vi "run.vi"(8 "error in (no error)":errorcluster, 11 "DL090503StimulatorScaffold in":refnum<class "StimulatorDL090503.lvclass">) -> (0 "error out":errorcluster, 3 "DL090503StimulatorScaffold out":refnum<class "StimulatorDL090503.lvclass">)   [LabVIEW 2010, in "StimulatorDL090503.lvclass"]
uses:
  StimulatorDL090503.lvclass
  pattern_type_enum.ctl
  common/xcontrols/XSettings/XSettings/XSettings.xctl
  common/classes/GenericComponent/GenericComponent/GenericComponent.lvclass
  main/labview_source/controls/undock_button.ctl
  StimulatorDL090503.lvclass/StimulatorDL090503.ctl
  StimulatorDL090503Scaffold/StimulatorDL090503Scaffold/StimulatorDL090503Scaffold.lvclass
  common/classes/ErrorController/ErrorController/class_data.vi
  GenericStimulator/GenericStimulator/GenericStimulator.lvclass
  common/classes/ErrorController/ErrorController/ErrorController.lvclass
panel:
  in  "button:undock":T1
  in  "Tab Control":enum32{"User", "Debug", "About"}(tab)
  in  "temp offset":dbl=1.0 caption="offset"
  in  "duration":dbl[unit]=1.0
  in  "test":bool
  in  "offset":dbl[unit]
  in  "repetition period":dbl[unit]=1.0
  in  "repetitions":i32=1
  out "stimulating?":bool
  in  "frequency":dbl[unit]=1.0
  in  "amplitude":dbl=1.0
  in  "XSettings":refnum<class "GenericComponent.lvclass">(xcontrol)
  in  "pattern":T2
  out "finished?":bool=TRUE
  out "loaded settings?":bool
  # "pattern"
  # "application"
  # "StimulatorDL090503\n\nImplemented by:\nDominik Langer, University of Zurich"
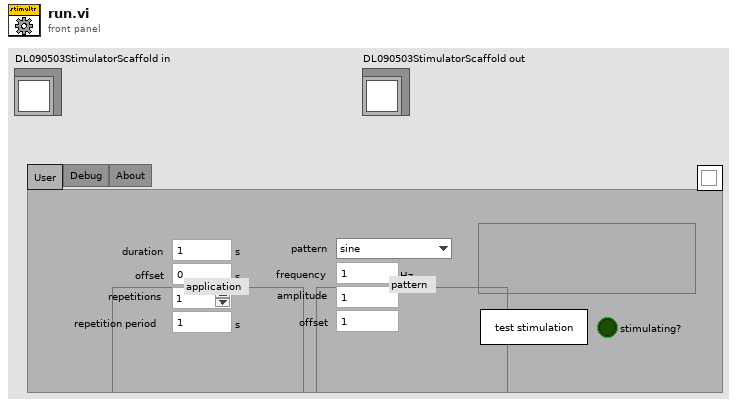
[diagram p1: front panel]
types:
  T1 = typedef "undock_button.ctl" = bool
  T2 = typedef "StimulatorDL090503.lvclass/pattern_type_enum.ctl" = enum16{"sine", "square (+/-)", "square (+)", "square (-)"}
  T3 = typedef "GenericToplevelComponent.lvclass/common_trigger_enum.ctl" = enum16{"NULL", "initialise", "terminate", "fetch command", "fetch data", "attach observer", "register as observer", "detach observer", "acknowledge", "start", "stop", "sweep started", "sweep finished", "experiment started", "experiment stopped"}
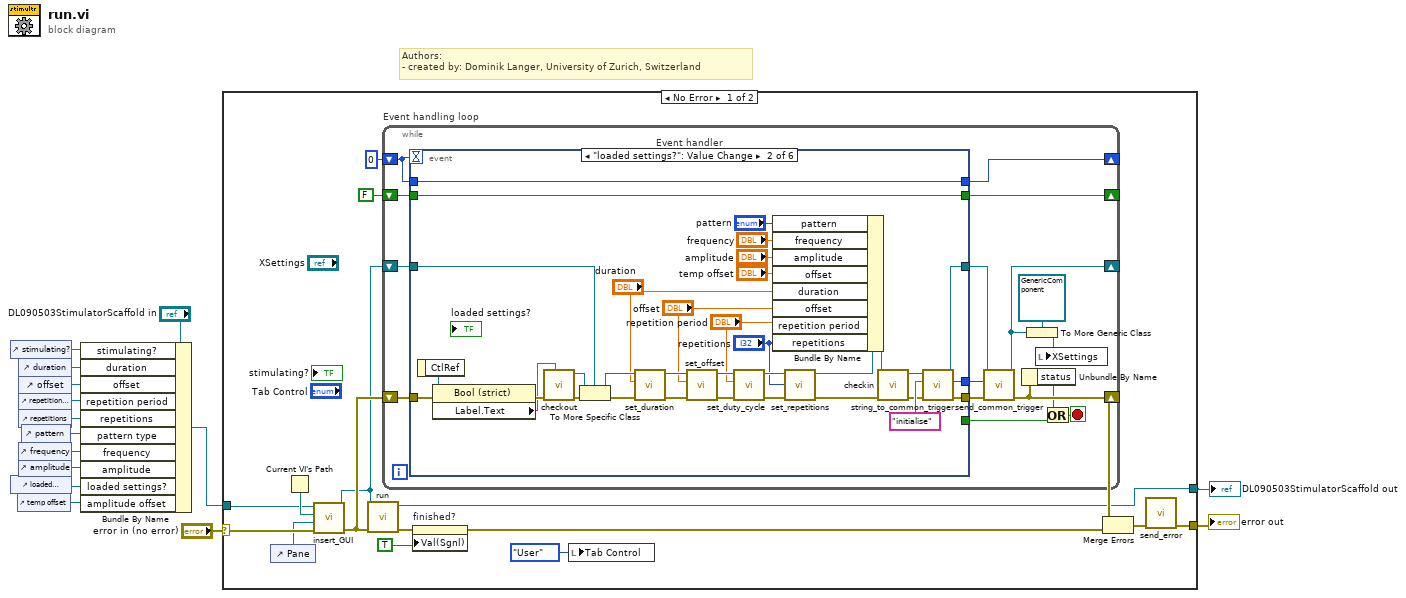
[diagram p0: block diagram]
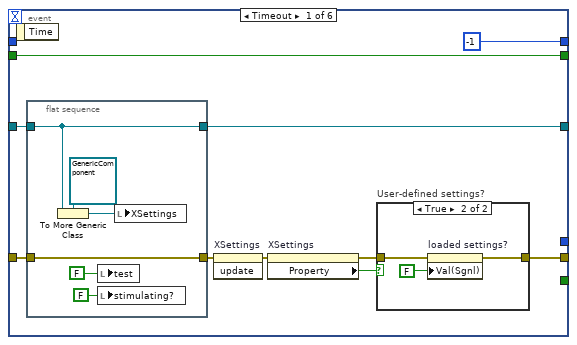
[diagram p2: hidden frame]
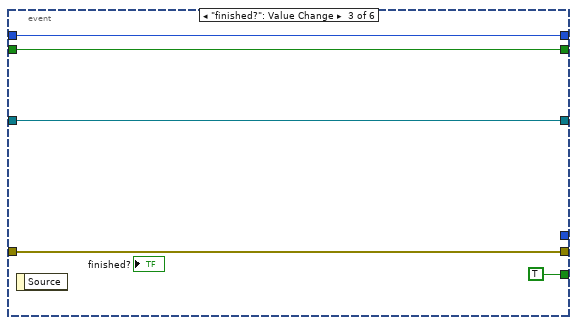
[diagram p4: hidden frame]
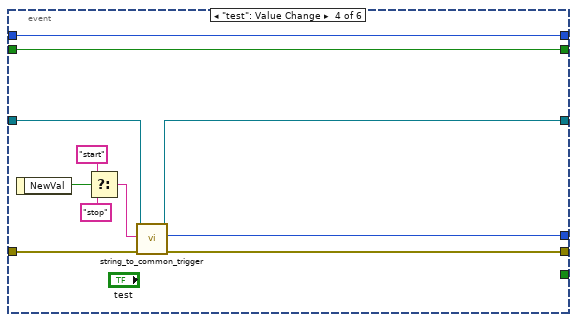
[diagram p5: hidden frame]
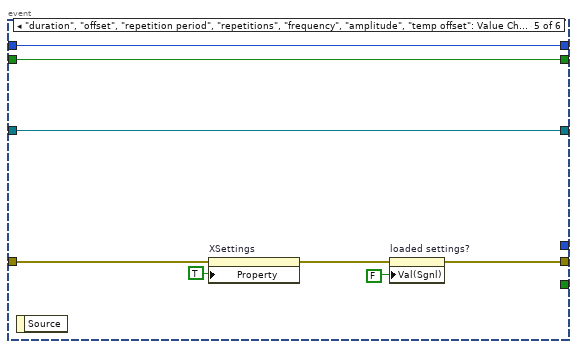
[diagram p6: hidden frame]
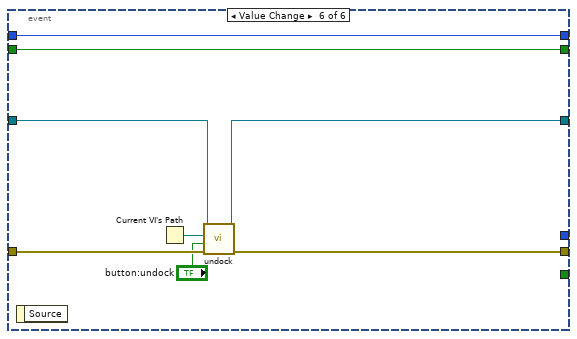
[diagram p7: hidden frame]
diagram:
  # "Authors: \n- created by: Dominik Langer, University of Zurich, Switzerland"
  n1 = control-ref of="stimulating?"() -> (w14:refnum<vi>)
  n2 = control-ref of="loaded settings?"() -> (w7:refnum<vi>)
  n3 = control-ref of="temp offset"() -> (w6:refnum<vi>)
  n4 = control-ref of="duration"() -> (w13:refnum<vi>)
  n5 = control-ref of="offset"() -> (w12:refnum<vi>)
  n6 = control-ref of="repetition period"() -> (w11:refnum<vi>)
  n7 = control-ref of="repetitions"() -> (w10:refnum<vi>)
  n8 = control-ref of="frequency"() -> (w9:refnum<vi>)
  n9 = control-ref of="amplitude"() -> (w8:refnum<vi>)
  n10 = control-ref of="pattern"() -> (w1:refnum<vi>)
  n11 = Bundle By Name(cluster="DL090503StimulatorScaffold in", "stimulating?"=w14, "duration"=w13, "offset"=w12, "repetition period"=w11, "repetitions"=w10, "pattern type"=w1, "frequency"=w9, "amplitude"=w8, "loaded settings?"=w7, "amplitude offset"=w6) -> (w15:refnum<class "StimulatorDL090503.lvclass">)
  n12 = case shown="No Error" "error in (no error)" {
    selector: "error in (no error)" -> [w22 w134]
    tunnel: [w18 w134] -> w4
    tunnel: w15 -> [w21 w135]
    tunnel: [w17 w135] -> w3
    frame No Error {
      n13 = control-ref of="Pane"() -> (w16:refnum<vi>)
      n14 = Current VI's Path() -> (path=w25:path)
      n15 = call-dynamic "insert_GUI.vi"("error in (no error)"=w22, "Pane"=w16, "VI path"=w25, "GenericComponent in"=w21) -> ("error out"=w26:errorcluster, "GenericComponent out"=w24:refnum<class "StimulatorDL090503.lvclass">)  [unwired: 6 in]
      n16 = call-parent "run.vi"("error in (no error)"=w26, "DL090503StimulatorScaffold in"=w24) -> ("error out"=w27:errorcluster, "DL090503StimulatorScaffold out"=w17:refnum<class "StimulatorDL090503.lvclass">)  [unwired: 8 out]
      n17 = while "Event handling loop" {
        shift-right: [w45] -> _
        shift-left: 0 -> [w46]
        shift-right: [w36] -> _
        shift-left: FALSE -> [w37]
        shift-right: [w41] -> w31
        shift-left: w26 -> [w47]
        shift-right: [w32] -> _
        shift-left: w24 -> [w44]
        stop <- w38 stop-if-true
        n18 = event "Event handler" shown="[1] \"loaded settings?\": Value Change" {
          selector: _ -> [_ _ _ _ _ _]
          dyn-events: _ -> [_ _ _ _ _ _]
          timeout: w46 -> [_ _ _ _ _ _]
          tunnel: w47 -> [w54 w98 w106 w114 w118 w131]
          tunnel: [w49 w76 w106 w113 w119 w130] -> w43
          tunnel: [_ _ TRUE _ _ _] -> w40
          tunnel: [-1 w101 w102 w117 w125 w133] -> w45
          tunnel: w46 -> [_ w101 w102 w117 w125 w133]
          tunnel: w44 -> [w55 w75 w104 w112 w122 w129]
          tunnel: [w53 w74 w104 w111 w122 w128] -> w34
          tunnel: [_ w71 _ w110 _ _] -> w42
          tunnel: w37 -> [w56 w100 w103 w116 w124 w132]
          tunnel: [w56 w100 w103 w116 w124 w132] -> w36
          event Timeout {
            n19 = event-data() -> ()  [unwired: 2 out]
            n20 = flat-sequence {
              tunnel: w55 -> [w63]
              tunnel: w54 -> [w62]
              tunnel: [w63] -> w53
              tunnel: [w62] -> w52
              frame #0 {
                n21 = To More Generic Class(target class=refnum<class "GenericComponent.lvclass"> refnum ("GenericComponent.lvclass"), reference=w63) -> (generic class reference=w65:refnum<class "GenericComponent.lvclass">)
                n22 = local write "test"(FALSE ("test")) -> ()
                n23 = local write "stimulating?"(FALSE ("stimulating?")) -> ()
                n24 = local write "XSettings"(w65) -> ()
              }
            }
            n25 = invoke on="XSettings" class="XSettings (strict)" method="update"(error in=w52) -> (error out=w51:errorcluster)  [unwired: 2 in, 2 out]
            n26 = property on="XSettings" class="XSettings (strict)"(error in=w51) -> (error out=w50:errorcluster, "Property"=w48:bool)  [unwired: 1 in, 1 out]
            n27 = case "User-defined settings?" shown="True" w48 {
              tunnel: w50 -> [w58 w60]
              tunnel: [w58 w59] -> w49
              frame False {
              }
              frame True {
                n28 = property on="loaded settings?" class="Bool (strict)"(error in=w60, "Val(Sgnl)"=FALSE) -> (error out=w59:errorcluster)  [unwired: 1 in, 1 out]
              }
            }
          }
          event "loaded settings?": Value Change {
            n29 = event-data() -> ("CtlRef"=w99:refnum<vi>)  [unwired: 1 out]
            n30 = property class="Bool (strict)"(reference=w99, error in=w98) -> (error out=w77:errorcluster, "Label.Text"=w72:string)  [unwired: 1 out]
            n31 = call "checkout.vi"("locked by?"=w72, "error in (no error)"=w77) -> ("error out"=w97:errorcluster, "GenericStimulator out"=w96:refnum<class "GenericStimulator.lvclass">)  [unwired: 8 out]
            n32 = To More Specific Class(target class=w75, reference=w96, error in=w97) -> (specific class reference=w95:refnum<class "StimulatorDL090503.lvclass">, error out=w94:errorcluster)
            n33 = call-dynamic "set_duration.vi"("error in (no error)"=w94, "duration"="duration", "DL090503StimulatorScaffold.lvclass in"=w95) -> ("error out"=w90:errorcluster, "DL090503StimulatorScaffold.lvclass out"=w88:refnum<class "StimulatorDL090503.lvclass">)  [unwired: 7 out]
            n34 = call-dynamic "set_offset.vi"("error in (no error)"=w90, "offset"="offset", "DL090503StimulatorScaffold.lvclass in"=w88) -> ("error out"=w89:errorcluster, "DL090503StimulatorScaffold.lvclass out"=w87:refnum<class "StimulatorDL090503.lvclass">)  [unwired: 7 out]
            n35 = call-dynamic "set_duty_cycle.vi"("error in (no error)"=w89, "duty cycle"="repetition period", "DL090503StimulatorScaffold.lvclass in"=w87) -> ("error out"=w92:errorcluster, "DL090503StimulatorScaffold.lvclass out"=w91:refnum<class "StimulatorDL090503.lvclass">)  [unwired: 7 out]
            n36 = call-dynamic "set_repetitions.vi"("error in (no error)"=w92, "repetitions"="repetitions", "DL090503StimulatorScaffold.lvclass in"=w91) -> ("error out"=w93:errorcluster, "DL090503StimulatorScaffold.lvclass out"=w82:refnum<class "StimulatorDL090503.lvclass">)  [unwired: 7 out]
            n37 = Bundle By Name(cluster=w82, "pattern"="pattern", "frequency"="frequency", "amplitude"="amplitude", "offset"="temp offset", "duration"="duration", "offset"="offset", "repetition period"="repetition period", "repetitions"="repetitions") -> (w81:refnum<class "StimulatorDL090503.lvclass">)
            n38 = call-dynamic "checkin.vi"("error in (no error)"=w93, "GenericStimulator in"=w81) -> ("error out"=w79:errorcluster, "GenericStimulator out"=w78:refnum<class "StimulatorDL090503.lvclass">)  [unwired: 8 in]
            n39 = call-dynamic "string_to_common_trigger.vi"("error in (no error)"=w79, "trigger string"="initialise", "GenericToplevelComponent in"=w78) -> ("error out"=w76:errorcluster, "trigger"=w71:T3, "GenericToplevelComponent out"=w74:refnum<class "StimulatorDL090503.lvclass">)  [unwired: 6 in]
          }
          event "finished?": Value Change {
            n40 = event-data() -> ()  [unwired: 2 out]
          }
          event "test": Value Change {
            n41 = event-data() -> ("NewVal"=w115:bool)  [unwired: 1 out]
            n42 = Select(t="start", s=w115, f="stop") -> (s? t:f=w109:string)
            n43 = call-dynamic "string_to_common_trigger.vi"("error in (no error)"=w114, "trigger string"=w109, "GenericToplevelComponent in"=w112) -> ("error out"=w113:errorcluster, "trigger"=w110:T3, "GenericToplevelComponent out"=w111:refnum<class "StimulatorDL090503.lvclass">)  [unwired: 6 in]
          }
          event "duration", "offset", "repetition period", "repetitions", "frequency", "amplitude", "temp offset": Value Change {
            n44 = event-data() -> ()  [unwired: 2 out]
            n45 = property on="XSettings" class="XSettings (strict)"(error in=w118, "Property"=TRUE ("is user-defined?")) -> (error out=w120:errorcluster)  [unwired: 1 in, 1 out]
            n46 = property on="loaded settings?" class="Bool (strict)"(error in=w120, "Val(Sgnl)"=FALSE) -> (error out=w119:errorcluster)  [unwired: 1 in, 1 out]
          }
          event Value Change {
            n47 = event-data() -> ()  [unwired: 2 out]
            n48 = Current VI's Path() -> (path=w126:path)
            n49 = call-dynamic "undock.vi"("error in (no error)"=w131, "undock?"="button:undock", "VI path"=w126, "GenericComponent in"=w129) -> ("error out"=w130:errorcluster, "GenericComponent out"=w128:refnum<class "StimulatorDL090503.lvclass">)  [unwired: 6 in]
          }
        }
        n50 = call-dynamic "send_common_trigger.vi"("error in (no error)"=w43, "trigger"=w42, "GenericToplevelComponent in"=w34) -> ("error out"=w41:errorcluster, "GenericToplevelComponent out"=w32:refnum<class "StimulatorDL090503.lvclass">)  [unwired: 6 in, 1 out]
        n51 = Unbundle By Name(w41) -> ("status"=w39:bool)
        n52 = To More Generic Class(target class=refnum<class "GenericComponent.lvclass"> refnum ("GenericComponent.lvclass"), reference=w32) -> (generic class reference=w35:refnum<class "GenericComponent.lvclass">)
        n53 = local write "XSettings"(w35) -> ()
        n54 = Or(x=w39, y=w40) -> (x .or. y?=w38:bool)
      }
      n55 = property on="finished?" class="Bool (strict)"(error in=w27, "Val(Sgnl)"=TRUE) -> (error out=w30:errorcluster)  [unwired: 1 in, 1 out]
      n56 = local write "Tab Control"(enum32{"User", "Debug", "About"}."User" ("Tab Control")) -> ()
      n57 = Merge Errors(w31, w30) -> (w19:errorcluster)
      n58 = call "send_error.vi"("error in (no error)"=w19) -> ("error out"=w18:errorcluster)  [unwired: 10 in]
    }
    frame Error {
    }
  }
  "error out" <- w4
  "DL090503StimulatorScaffold out" <- w3
